vi "toXML.vi"(8 "error in (no error)":errorcluster, 11 "Loop in":refnum<class "Loop.lvclass">) -> (0 "error out":errorcluster, 2 "xmlNode":refnum<class "xmlNode.lvclass">, 3 "Loop out":refnum<class "Loop.lvclass">)   [LabVIEW 2009, in "Tools.lvlib" / "Sequencing.lvlib" / "Loop.lvclass"]
uses:
  Loop.lvclass
  xmlNode/xmlNode.lvclass
  Loop.lvclass/Loop.ctl
  Point/Point.lvclass
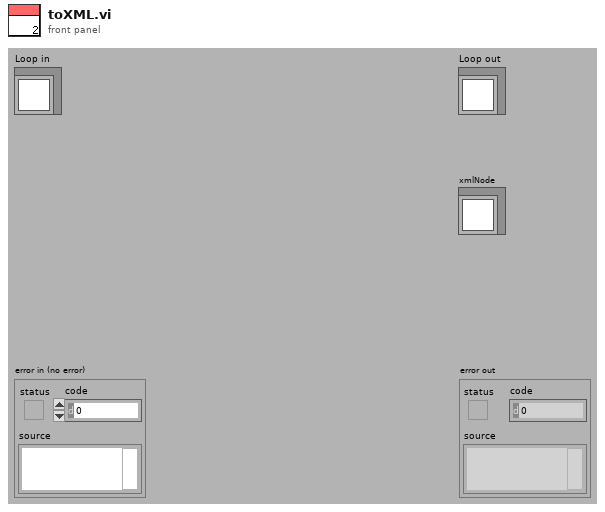
[diagram p1: front panel]
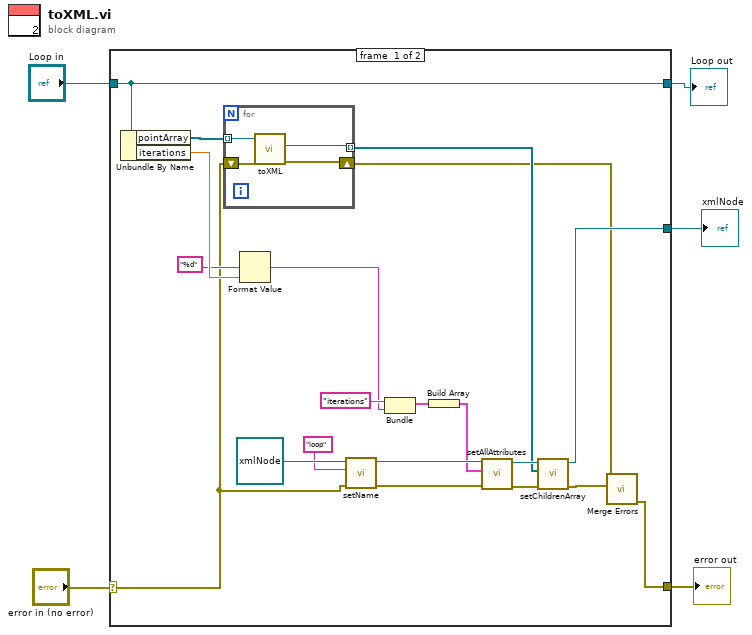
[diagram p0: block diagram]
diagram:
  n1 = case shown="No Error" "error in (no error)" {
    selector: "error in (no error)" -> [w13 w30]
    tunnel: [w25 w31] -> w5
    tunnel: "Loop in" -> [w25 w31]
    tunnel: [w6 w30] -> w2
    tunnel: [w9 _] -> w1
    frame #0 {
      n2 = Unbundle By Name(w25) -> ("pointArray"=w24:refnum<class "Point.lvclass">[], "iterations"=w19:dbl)
      n3 = for {
        tunnel: w24 -> [w29] mode=indexing
        tunnel: [w28] -> w10 mode=indexing
        shift-right: [w26] -> w8
        shift-left: w13 -> [w27]
        n4 = call-parent "toXML.vi"("error in (no error)"=w27, "Point in"=w29) -> ("error out"=w26:errorcluster, "xmlNode"=w28:refnum<class "xmlNode.lvclass">)  [unwired: 7 in, 1 out]
      }
      n5 = Format Value(format string="%d", value (0)=w19) -> (output string=w16:string)  [unwired: 1 in]
      n6 = call-dynamic "setName.vi"("error in (no error)"=w13, "name"="loop", "xmlNode.lvclass in"=refnum<class "xmlNode.lvclass"> refnum ("Tools.lvlib:xml.lvlib:xmlNode.lvclass")) -> ("error out"=w20:errorcluster, "xmlNode.lvclass out"=w21:refnum<class "xmlNode.lvclass">)  [unwired: 7 in]
      n7 = Bundle("iterations", "output string"=w16) -> (w15:cluster{string, "output string":string})  [unwired: 1 in]
      n8 = Build Array(w15) -> (w14:cluster{string, "output string":string}[])
      n9 = call-dynamic "setAllAttributes.vi"("error in (no error)"=w20, "attributes"=w14, "xmlNode in"=w21) -> ("error out"=w11:errorcluster, "xmlNode out"=w12:refnum<class "xmlNode.lvclass">)  [unwired: 7 in]
      n10 = call-dynamic "setChildrenArray.vi"("error in (no error)"=w11, "Children"=w10, "xmlNode.lvclass in"=w12) -> ("error out"=w7:errorcluster, "xmlNode.lvclass out"=w9:refnum<class "xmlNode.lvclass">)  [unwired: 7 in]
      n11 = call <vilib>:"Merge Errors.vi"("error in 2 (no error)"=w7, "error in 1 (no error)"=w8) -> ("error out"=w6:errorcluster)  [unwired: 5 in]
    }
    frame #1 {
    }
  }
  "error out" <- w2
  "Loop out" <- w5
  "xmlNode" <- w1
